vi "Server.vi"() -> ()   [LabVIEW 2021]
panel:
  in  "stop":bool
  in  "Tamper":cluster{u32, u32}[](array[cluster])
  in  "Bypass":cluster{u32, u32}[](array[cluster])
  in  "Alarm":cluster{u32, u32}[](array[cluster])
  in  "Normal":cluster{u32, u32}[](array[cluster])
  out "Zone 1":bool
  # "Green: Normal\nRed: Alarm\nBlue:Bypass\nOrange: Tamper"
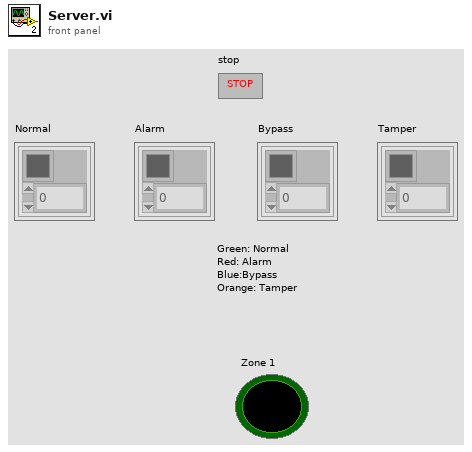
[diagram p1: front panel]
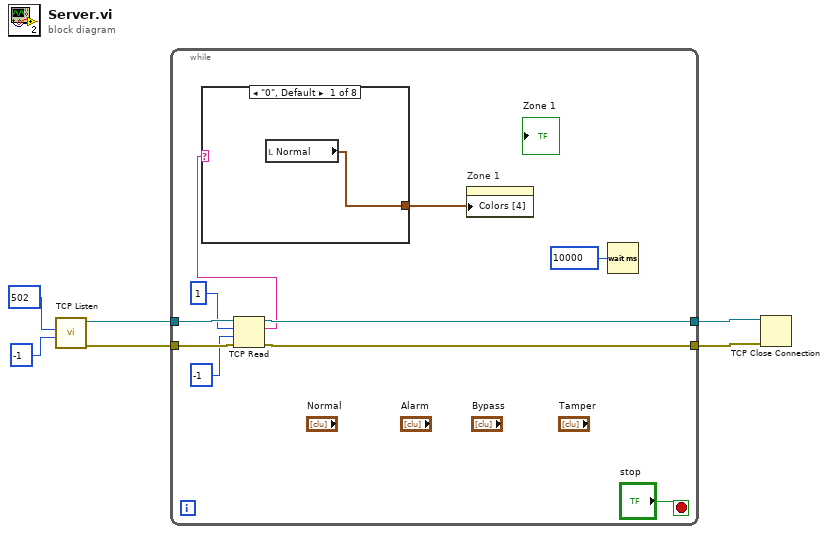
[diagram p0: block diagram]
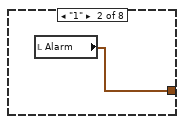
[diagram p2: hidden frame]
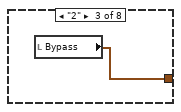
[diagram p3: hidden frame]
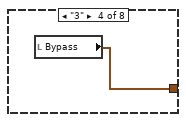
[diagram p4: hidden frame]
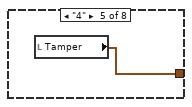
[diagram p5: hidden frame]
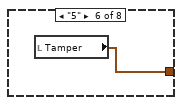
[diagram p6: hidden frame]
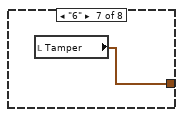
[diagram p7: hidden frame]
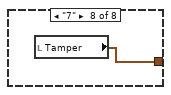
[diagram p8: hidden frame]
diagram:
  n1 = call <vilib>:"TCP Listen.vi"("timeout ms (wait forever: -1)"=-1, "port"=u16 502) -> ("error out"=w3:errorcluster, "connection ID"=w4:refnum<k5>)  [unwired: 5 in, 3 out]
  n2 = while {
    tunnel: w4 -> [w16]
    tunnel: w3 -> [w15]
    tunnel: [w14] -> w2
    tunnel: [w13] -> w1
    stop <- "stop" stop-if-true
    n3 = TCP Read(connection ID=w16, bytes to read=1, error in (no error)=w15, 9:-1 ("timeout ms (25000)")) -> (connection ID out=w14:refnum<k5>, data out=w10:string, error out=w13:errorcluster)  [unwired: 1 in]
    n4 = case shown="\"0\", Default" w10 {
      tunnel: [w17 w18 w19 w20 w21 w22 w23 w24] -> w9
      frame "0", Default {
        n5 = local read "Normal"() -> (w17:cluster{u32, u32}[])
      }
      frame "1" {
        n6 = local read "Alarm"() -> (w18:cluster{u32, u32}[])
      }
      frame "2" {
        n7 = local read "Bypass"() -> (w19:cluster{u32, u32}[])
      }
      frame "3" {
        n8 = local read "Bypass"() -> (w20:cluster{u32, u32}[])
      }
      frame "4" {
        n9 = local read "Tamper"() -> (w21:cluster{u32, u32}[])
      }
      frame "5" {
        n10 = local read "Tamper"() -> (w22:cluster{u32, u32}[])
      }
      frame "6" {
        n11 = local read "Tamper"() -> (w23:cluster{u32, u32}[])
      }
      frame "7" {
        n12 = local read "Tamper"() -> (w24:cluster{u32, u32}[])
      }
    }
    n13 = property on="Zone 1" class="Bool (strict)"("Colors [4]"=w9) -> ()  [unwired: 2 in, 2 out]
    n14 = Wait (ms)(milliseconds to wait=u32 10000) -> ()  [unwired: 1 out]
  }
  n15 = TCP Close Connection(connection ID=w2, error in (no error)=w1) -> ()  [unwired: 1 in, 2 out]
